vi "Handle Error.vi"(8 "error in (no error)":errorcluster, 11 "AF IMAQ Display in":refnum<class "HIJ Vision Display.lvclass">) -> (0 "error out":errorcluster, 2 "stop actor?":bool=TRUE, 3 "AF IMAQ Display out":refnum<class "HIJ Vision Display.lvclass">)   [LabVIEW 2014, in "HIJ Vision Display.lvlib" / "HIJ Vision Display.lvclass"]
doc: "(<B>Filename</B>: Actor Framework.lvlib:Actor.lvclass:Handle Error.vi)\n\nDefines how the actor handles an error that occurred while processing a message. By default, this method does nothing except stop the actor."
uses:
  HIJ Vision Display.lvclass
  Shared Code/Viewable Actor/ViewableActor/ViewableActor.lvclass
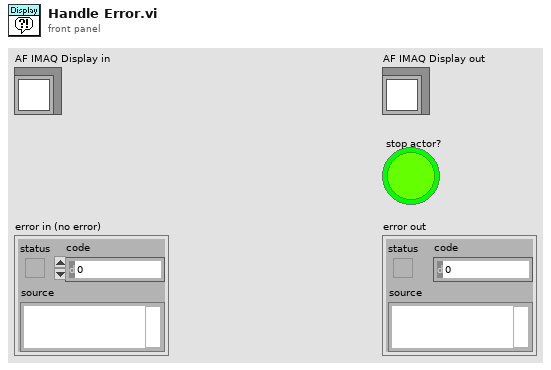
[diagram p1: front panel]
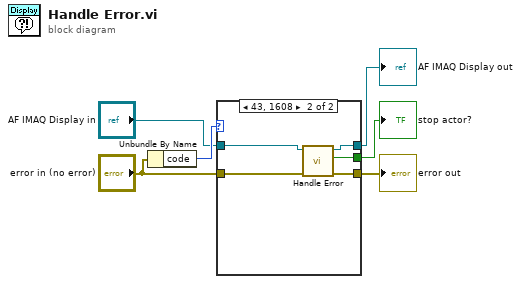
[diagram p0: block diagram]
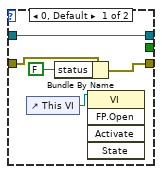
[diagram p2: hidden frame]
diagram:
  n1 = Unbundle By Name("error in (no error)") -> ("code"=w6:i32)
  n2 = case shown="43, 1608" w6 {
    tunnel: [w10 w16] -> w2
    tunnel: [_ w15] -> w1
    tunnel: [w8 w14] -> w3
    tunnel: "error in (no error)" -> [w11 w13]
    tunnel: "AF IMAQ Display in" -> [w8 w12]
    frame 0, Default {
      n3 = control-ref of="This VI"() -> (w7:refnum<vi>)
      n4 = Bundle By Name(cluster=w11, "status"=FALSE) -> (w10:errorcluster)
      n5 = invoke class="VI" method="FP.Open"(reference=w7) -> ()  [unwired: 4 in, 5 out]
    }
    frame 43, 1608 {
      n6 = call-parent "Handle Error.vi"("error in (no error)"=w13, "Actor in"=w12) -> ("error out"=w16:errorcluster, "stop actor?"=w15:bool, "Actor out"=w14:refnum<class "HIJ Vision Display.lvclass">)  [unwired: 7 in]
    }
  }
  "AF IMAQ Display out" <- w3
  "error out" <- w2
  "stop actor?" <- w1
